vi "Get Temperature DBL.vi"(8 "error in":errorcluster, 10 "Source":string, 11 "Thermometer Multichannel Worker in":refnum<class "Thermometer Multichannel Worker.lvclass">) -> (0 "error out":errorcluster, 1 "Time Stamp":timestamp format="%<%x %.3X>T", 2 "Temperature":dbl, 3 "Thermometer Multichannel Worker out":refnum<class "Thermometer Multichannel Worker.lvclass">)   [LabVIEW 2024, in "Thermometer Multichannel Worker.lvlib" / "Thermometer Multichannel Worker.lvclass"]
uses:
  Thermometer Multichannel Worker.lvclass
  Thermometer Multichannel Worker.lvclass/Thermometer Multichannel Worker.ctl
  <vilib>/Waveform/WDTOps.llb/WDT Get Final Time Value DBL.vi
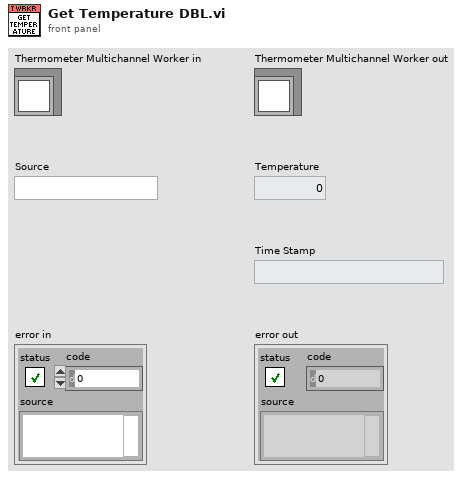
[diagram p1: front panel]
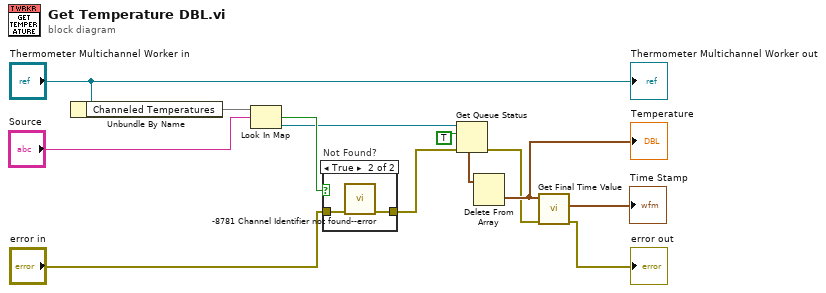
[diagram p0: block diagram]
diagram:
  n1 = Unbundle By Name("Thermometer Multichannel Worker in") -> ("Channeled Temperatures"=w12:map{string, refnum<queue>})
  n2 = Look In Map(map=w12, key="Source") -> (key not found?=w9:bool, value=w8:refnum<queue>)  [unwired: 1 in]
  n3 = case "Not Found?" shown="True" w9 {
    tunnel: [w14 w16] -> w7
    tunnel: "error in" -> [w14 w15]
    frame False {
    }
    frame True {
      n4 = call "-8781 Channel Identifier not found--error.vi"("error in"=w15) -> ("error out"=w16:errorcluster)  [unwired: 10 in]
    }
  }
  n5 = Get Queue Status(queue=w8, return elements? (F)=TRUE, error in (no error)=w7) -> (error out=w1:errorcluster, elements=w5:waveform(dbl)[])  [unwired: 6 out]
  n6 = Delete From Array(array=w5) -> (deleted portion=w4:waveform(dbl))  [unwired: 2 in, 1 out]
  "Temperature" <- w4
  n7 = call-poly <vilib>:"Get Final Time Value.vi"("error in (no error)"=w1, "waveform in"=w4) -> ("error out"=→"error out":errorcluster, "tf"=→"Time Stamp":timestamp)  [unwired: 7 in, 1 out]
  "Thermometer Multichannel Worker out" <- "Thermometer Multichannel Worker in"
